vi "input.vi"(8 "error in":errorcluster, 10 "data table in":T1, 11 "TEC runtime in":refnum<class "TEC runtime.lvclass">) -> (0 "error out":errorcluster, 2 "data table out":T1, 3 "TEC runtime out":refnum<class "TEC runtime.lvclass">)   [LabVIEW 2013, in "TEC runtime.lvclass"]
doc: "Provides an interface for reading data from a module at runtime. While this interface performs no operations, a child should provide an override which may read from any open sessions, references, or interfaces."
uses:
  TEC runtime.lvclass
  <vilib>/NI/Tag Bus/table/data table.ctl
  TEC runtime.lvclass/TEC runtime.ctl
  <vilib>/NI/Current Value Table/Read Index Set.vi
  <vilib>/NI/Current Value Table/DataTypes/Double_Read Index Set.vi
  <vilib>/NI/Current Value Table/DataTypes/Array of String_Read Index Set.vi
  <vilib>/NI/Current Value Table/DataTypes/Array of Boolean_Read Index Set.vi
  <vilib>/NI/Current Value Table/DataTypes/Array of Single_Read Index Set.vi
  <vilib>/NI/Current Value Table/DataTypes/Array of Double_Read Index Set.vi
  <vilib>/NI/Current Value Table/DataTypes/Array of I8_Read Index Set.vi
  <vilib>/NI/Current Value Table/DataTypes/Array of I16_Read Index Set.vi
  <vilib>/NI/Current Value Table/DataTypes/Array of I32_Read Index Set.vi
  <vilib>/NI/Current Value Table/DataTypes/Array of I64_Read Index Set.vi
  <vilib>/NI/Current Value Table/DataTypes/Array of U64_Read Index Set.vi
  <vilib>/NI/Current Value Table/DataTypes/Array of U32_Read Index Set.vi
  <vilib>/NI/Current Value Table/DataTypes/Array of U16_Read Index Set.vi
  <vilib>/NI/Current Value Table/DataTypes/Array of U8_Read Index Set.vi
  <vilib>/NI/Current Value Table/DataTypes/Boolean_Read Index Set.vi
  <vilib>/NI/Current Value Table/DataTypes/String_Read Index Set.vi
  <vilib>/NI/Current Value Table/DataTypes/U8_Read Index Set.vi
  <vilib>/NI/Current Value Table/DataTypes/U16_Read Index Set.vi
  <vilib>/NI/Current Value Table/DataTypes/U32_Read Index Set.vi
  <vilib>/NI/Current Value Table/DataTypes/U64_Read Index Set.vi
  <vilib>/NI/Current Value Table/DataTypes/I8_Read Index Set.vi
  <vilib>/NI/Current Value Table/DataTypes/I16_Read Index Set.vi
  <vilib>/NI/Current Value Table/DataTypes/I32_Read Index Set.vi
  <vilib>/NI/Current Value Table/DataTypes/I64_Read Index Set.vi
  <vilib>/NI/Current Value Table/DataTypes/Single_Read Index Set.vi
  <vilib>/NI/Current Value Table/Memory Block.vi
  <vilib>/NI/Current Value Table/DataTypes/Double_Memory Block.vi
  <vilib>/NI/Current Value Table/DataTypes/Array of String_Memory Block.vi
  <vilib>/NI/Current Value Table/DataTypes/Array of Boolean_Memory Block.vi
  <vilib>/NI/Current Value Table/DataTypes/Array of Single_Memory Block.vi
  <vilib>/NI/Current Value Table/DataTypes/Array of Double_Memory Block.vi
  <vilib>/NI/Current Value Table/DataTypes/Array of I8_Memory Block.vi
  <vilib>/NI/Current Value Table/DataTypes/Array of I16_Memory Block.vi
  <vilib>/NI/Current Value Table/DataTypes/Array of I32_Memory Block.vi
  <vilib>/NI/Current Value Table/DataTypes/Array of I64_Memory Block.vi
  <vilib>/NI/Current Value Table/DataTypes/Array of U64_Memory Block.vi
  <vilib>/NI/Current Value Table/DataTypes/Array of U32_Memory Block.vi
  <vilib>/NI/Current Value Table/DataTypes/Array of U16_Memory Block.vi
  <vilib>/NI/Current Value Table/DataTypes/Array of U8_Memory Block.vi
  <vilib>/NI/Current Value Table/DataTypes/Boolean_Memory Block.vi
  <vilib>/NI/Current Value Table/DataTypes/String_Memory Block.vi
  <vilib>/NI/Current Value Table/DataTypes/U8_Memory Block.vi
  <vilib>/NI/Current Value Table/DataTypes/U16_Memory Block.vi
  <vilib>/NI/Current Value Table/DataTypes/U32_Memory Block.vi
  <vilib>/NI/Current Value Table/DataTypes/U64_Memory Block.vi
  <vilib>/NI/Current Value Table/DataTypes/I8_Memory Block.vi
  <vilib>/NI/Current Value Table/DataTypes/I16_Memory Block.vi
  <vilib>/NI/Current Value Table/DataTypes/I32_Memory Block.vi
  <vilib>/NI/Current Value Table/DataTypes/I64_Memory Block.vi
  <vilib>/NI/Current Value Table/DataTypes/Single_Memory Block.vi
  <vilib>/NI/Tag Bus/table/data table.lvlib
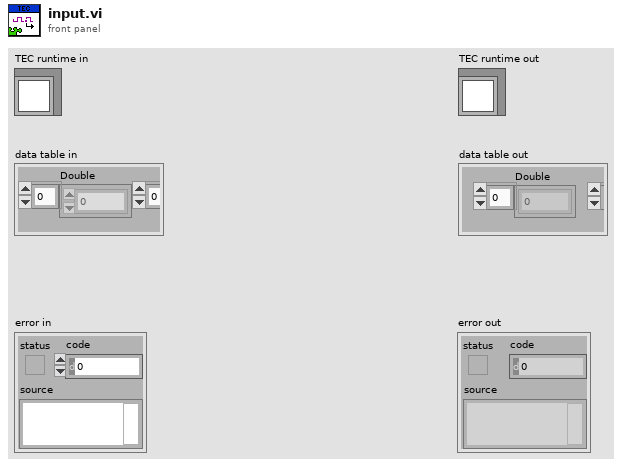
[diagram p1: front panel]
types:
  T1 = typedef "tag bus.lvlib/data table.lvlib/data table.ctl" = cluster{"Double":dbl[], "Single":sgl[], "I64":i64[], "I32":i32[], "I16":i16[], "I8":i8[], "U64":u64[], "U32":u32[], "U16":u16[], "U8":u8[], "Boolean":bool[], "String":string[], "Array of Double":cluster{"DBL Array":dbl[]}[], "Array of Single":cluster{"SGL Array":sgl[]}[], "Array of I64":cluster{"I64 Array":i64[]}[], "Array of I32":cluster{"I32 Array":i32[]}[], "Array of I16":cluster{"I16 Array":i16[]}[], "Array of I8":cluster{"I8 Array":i8[]}[], "Array of U64":cluster{"U64 Array":u64[]}[], "Array of U32":cluster{"U32 Array":u32[]}[], "Array of U16":cluster{"U16 Array":u16[]}[], "Array of U8":cluster{"U8 Array":u8[]}[], "Array of Boolean":cluster{"Boolean Array":bool[]}[], "Array of String":cluster{"String Array":string[]}[]}
  T2 = typedef "Current Value Table.lvlib/Typed Index Set.ctl" = cluster{"Data Type":T3, "Indices":i32[]}
  T3 = typedef "Current Value Table.lvlib/Data Types.ctl" = enum16{"Double", "Single", "I64", "I32", "I16", "I8", "U64", "U32", "U16", "U8", "String", "Boolean", "Array of U8", "Array of U16", "Array of U32", "Array of U64", "Array of I64", "Array of I32", "Array of I16", "Array of I8", "Array of Double", "Array of Single", "Array of Boolean", "Array of String"}
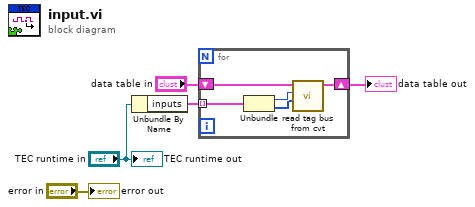
[diagram p0: block diagram]
diagram:
  n1 = Unbundle By Name("TEC runtime in") -> ("inputs"=w4:T2[])
  n2 = for {
    tunnel: w4 -> [w10] mode=indexing
    shift-right: [w9] -> w2
    shift-left: "data table in" -> [w8]
    n3 = Unbundle(w10) -> ("Data Type"=w7:T3, "Indices"=w6:i32[])
    n4 = call "read tag bus from cvt.vi"("Indices"=w6, "Data Type"=w7, "data table in"=w8) -> ("data table out"=w9:T1)  [unwired: 8 in]
  }
  "data table out" <- w2
  "error out" <- "error in"
  "TEC runtime out" <- "TEC runtime in"
